vi "Calculate ENBW RC.vi"(10 "filter order":i32, 11 "time constant (s)":dbl) -> (3 "ENBW (Hz)":dbl)   [LabVIEW 2019, in "DSP.lvclass"]
uses:
  DSP.lvclass
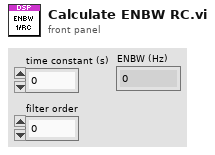
[diagram p1: front panel]
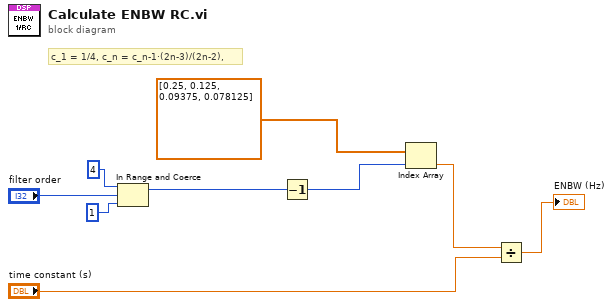
[diagram p0: block diagram]
diagram:
  # "c_1 = 1/4, c_n = c_n-1·(2n-3)/(2n-2),"
  n1 = In Range and Coerce(upper limit=4 ("lower limit"), x="filter order", lower limit=1) -> (coerced(x)=w3:i32)  [unwired: 1 out]
  n2 = Decrement(x=w3) -> (x-1=w2:i32)
  n3 = Index Array(array=dbl[] [0.25, 0.125, 0.09375, 0.078125], index=w2) -> (element=w1:dbl)
  n4 = Divide(x=w1, y="time constant (s)") -> (x/y=→"ENBW (Hz)":dbl)
